vi "Strlen.vi"(7 "Check Size Limit (F)":bool, 8 "No Error":errorcluster, 11 "Str [const char *]":i64 format="%.0x") -> (0 "Error Out":errorcluster, 3 "Size":u64)   [LabVIEW 2026, in "SDL3.lvlib" / "Stdinc.lvlib"]
doc: "<B>Summary</B>\nThis works exactly like strlen() but doesn't require access to a C runtime.\n\n<B>Remarks</B>\nCounts the bytes in str, excluding the null terminator.\n\nIf you need the length of a UTF-8 string, consider using <B>SDL_utf8strlen()</B>."
uses:
  Stdinc.lvlib
  c3f57b18-2899-4d18-8de7-ed42e0d99649.vi
  Lib/SDL3.dll
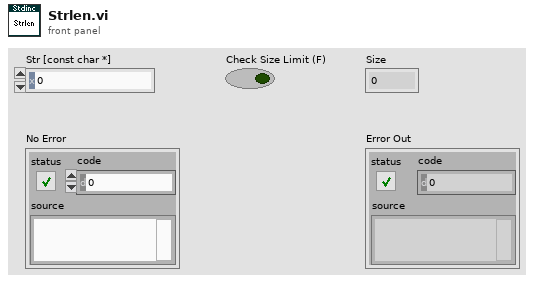
[diagram p1: front panel]
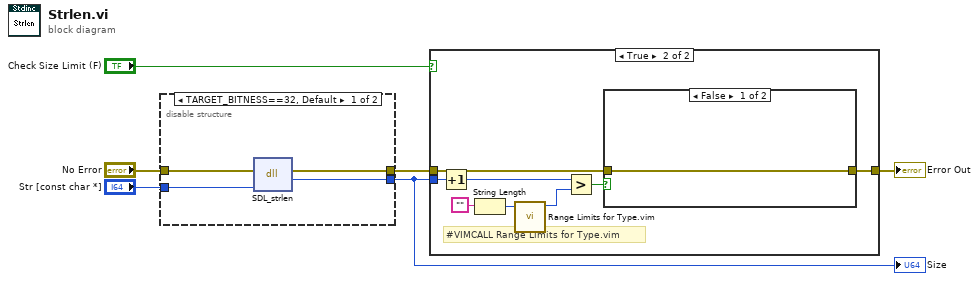
[diagram p0: block diagram]
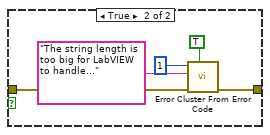
[diagram p3: hidden frame]
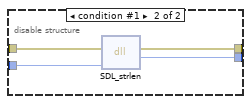
[diagram p4: hidden frame]
diagram:
  n1 = disable-structure shown="TARGET_BITNESS==32, Default" {
    disable-tunnel: "Str [const char *]" -> [w10 w14]
    disable-tunnel: "No Error" -> [w9 w13]
    disable-tunnel: [w8 w12] -> w4
    disable-tunnel: [w7 w11] -> w3
    frame condition #0 (active) {
      n2 = dll-call lib="C:/Users/saukko/Dev/LV-SDL3/Sources/SDL3/Lib/SDL3.*" fn="SDL_strlen"(error in=w9, "str"=w10) -> (error out=w8:errorcluster, "return type"=w7:u32)  [unwired: 3 in, 1 out]
    }
    frame condition #1 {
      n3 = dll-call lib="C:/Users/saukko/Dev/LV-SDL3/Sources/SDL3/Lib/SDL3.*" fn="SDL_strlen"(error in=w13, "str"=w14) -> (error out=w12:errorcluster, "return type"=w11:u64)  [unwired: 3 in, 1 out]
    }
  }
  "Size" <- w3
  n4 = case shown="True" "Check Size Limit (F)" {
    tunnel: w4 -> [w15 w23]
    tunnel: w3 -> [_ w22]
    tunnel: [w15 w21] -> w2
    frame False {
    }
    frame True {
      # "#VIMCALL Range Limits for Type.vim"
      n5 = Increment(x=w22) -> (x+1=w18:u32)
      n6 = String Length(string="") -> (length=w17:i32)
      n7 = call "Range Limits for Type.vim"("type"=w17) -> ("maximum value for type"=w16:i32)  [unwired: 9 in, 1 out]
      n8 = Greater?(x=w18, y=w16) -> (0:w20:bool)
      n9 = case shown="False" w20 {
        tunnel: w23 -> [w24 w29]
        tunnel: [w24 w28] -> w21
        frame False {
        }
        frame True {
          n10 = call <vilib>:"Error Cluster From Error Code.vi"("show call chain? (False)"=TRUE, "error in (no error)"=w29, "error message (\"\")"="The string length is too big for LabVIEW to handle..." ("error message (\"\")"), "error code (0)"=1) -> ("error out"=w28:errorcluster)  [unwired: 5 in]
        }
      }
    }
  }
  "Error Out" <- w2
